vi "Alarm Settings.vi"(3 "Avg Temp Alarm On?":bool) -> (0 "Array of alarm limits":i32[](array[numeric]))   [LabVIEW 2014]
uses:
  <vilib>/Platform/TimedLoop/XDataNode/XDataNode.xnode
  <vilib>/Platform/TimedLoop/XDataNode/nitl_modes.ctl
  <vilib>/Platform/TimedLoop/XDataNode/XDNodeRunTimeDep.lvlib
  <vilib>/Platform/TimedLoop/XDataNode/wakeup.ctl
  <vilib>/Platform/TimedLoop/XDataNode/timing_clust.ctl
panel:
  in  "Max Spike":i32
  in  "Temperature Bounds High":i32
  in  "Temperature Bounds Low":i32
  # "Alarm Settings"
  # "Low"
  # "High"
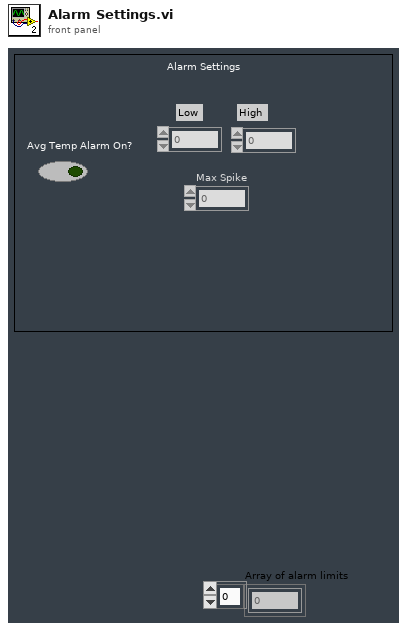
[diagram p1: front panel]
types:
  T1 = typedef "XDNodeRunTimeDep.lvlib/timing_clust.ctl" = cluster{"Expected End [f-1]":u64, "Actual End [f-1]":u64, "Finished Late? [f-1]":bool, "Expected End [i-1]":u64, "Actual End [i-1]":u64, "Finished Late? [i-1]":bool, "Expected Start [i]":u64, "Actual Start [i]":u64, "Expected Start [f]":u64, "Actual Start [f]":u64, "Source Name":string, "Structure Name":string, "Period":i64, "Deadline":i64, "Offset":i64, "Start":i64, "Priority":i32, "Timeout":i32, "Mode":T2, "Wakeup Reason":T3, "Error":errorcluster, "Source Type":string, "Secondary Source Type":string, "Global End Time":u64, "Global Start Time":u64, "Frame Duration":u64, "Iteration Duration":u64, "Assigned CPU":i32, "I/O Scan Engine Mode":u32}
  T2 = typedef "XDNodeRunTimeDep.lvlib/nitl_modes.ctl" = enum32{"No Change", "Process missed periods, maintain original phase", "Discard missed periods, maintain original phase", "Process missed periods, ignore original phase", "Discard missed periods, ignore original phase"}
  T3 = typedef "XDNodeRunTimeDep.lvlib/wakeup.ctl" = enum32{"Normal", "Aborted", "Asynchronous wakeup", "Timing source error", "Timed loop error", "Timeout"}
  T4 = enum8{"Enabled", "Disabled", "Disabled and Grayed Out"}
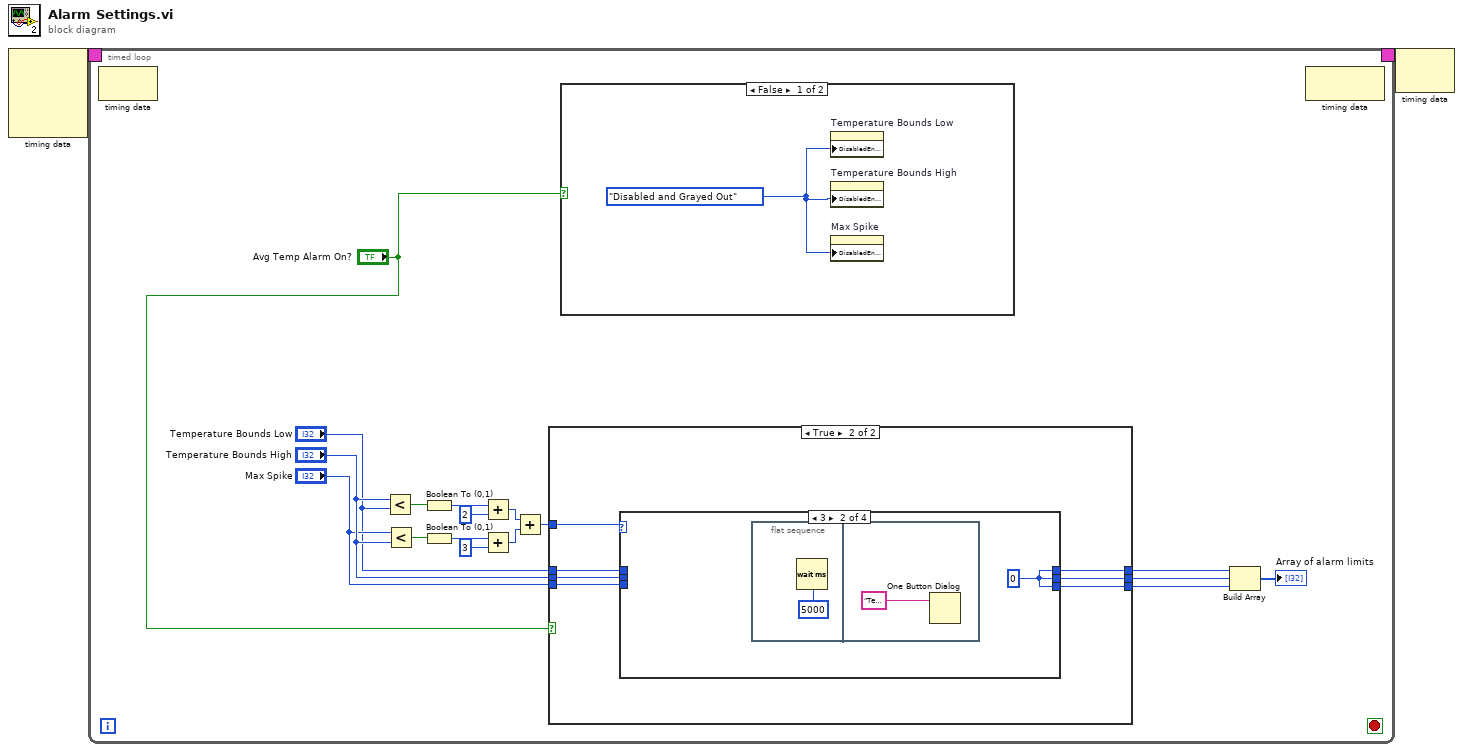
[diagram p0: block diagram]
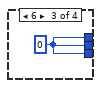
[diagram p4: hidden frame]
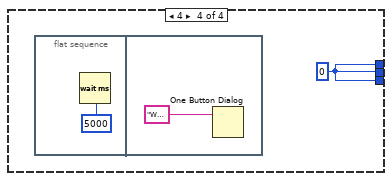
[diagram p5: hidden frame]
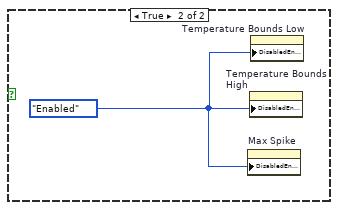
[diagram p6: hidden frame]
diagram:
  n1 = node-c288() -> (w2:T1)  [unwired: 4 in]
  n2 = timed-loop {
    timing: w2 -> [_]
    timing-out: [_] -> w1
    stop <- _ stop-if-true
    n3 = node-c288() -> ()  [unwired: 1 in, 1 out]
    n4 = Less?(x="Temperature Bounds High", y="Temperature Bounds Low") -> (x < y?=w16:bool)
    n5 = Less?(x="Max Spike", y="Temperature Bounds High") -> (x < y?=w11:bool)
    n6 = Boolean To (0,1)(Boolean=w16) -> (0, 1=w15:i16)
    n7 = Boolean To (0,1)(Boolean=w11) -> (0, 1=w13:i16)
    n8 = Add(x=w15, y=i16 2) -> (x+y=w9:i16)
    n9 = Add(x=w13, y=i16 3) -> (x+y=w10:i16)
    n10 = Add(x=w9, y=w10) -> (x+y=w8:i16)
    n11 = case shown="True" "Avg Temp Alarm On?" {
      tunnel: "Temperature Bounds High" -> [_ w22]
      tunnel: w8 -> [_ w26]
      tunnel: [_ w25] -> w7
      tunnel: [_ w24] -> w6
      tunnel: [_ w23] -> w5
      tunnel: "Max Spike" -> [_ w21]
      tunnel: "Temperature Bounds Low" -> [_ w20]
      frame False {
      }
      frame True {
        n12 = case shown="3" w26 {
          tunnel: [w27 w30 w33 w34] -> w25
          tunnel: [w29 w30 w33 w34] -> w24
          tunnel: [w28 w30 w33 w34] -> w23
          tunnel: w22 -> [w29 _ _ _]
          tunnel: w21 -> [w28 _ _ _]
          tunnel: w20 -> [w27 _ _ _]
          frame 5, Default {
          }
          frame 3 {
            w30 = 0 ("Temperature Bounds High")
            n13 = flat-sequence {
              frame #0 {
                n14 = Wait (ms)(milliseconds to wait=u32 5000) -> ()  [unwired: 1 out]
              }
              frame #1 {
                n15 = One Button Dialog(message="Temperature minimum higher than Temperature maximum!ARNING: Max Spike must be set higher than the Max Temperature Bounds!") -> ()  [unwired: 1 in, 1 out]
              }
            }
          }
          frame 6 {
            w33 = 0
          }
          frame 4 {
            w34 = 0 ("Temperature Bounds High")
            n16 = flat-sequence {
              frame #0 {
                n17 = Wait (ms)(milliseconds to wait=u32 5000) -> ()  [unwired: 1 out]
              }
              frame #1 {
                n18 = One Button Dialog(message="WARNING: Max Spike must be set higher than the Max Temperature Bounds!") -> ()  [unwired: 1 in, 1 out]
              }
            }
          }
        }
      }
    }
    n19 = case shown="False" "Avg Temp Alarm On?" {
      frame False {
        w39 = T4."Disabled and Grayed Out" ("Disabled")
        n20 = property on="Temperature Bounds Low" class="DigNum (strict)"("DisabledEnum"=w39) -> ()  [unwired: 2 in, 2 out]
        n21 = property on="Temperature Bounds High" class="DigNum (strict)"("DisabledEnum"=w39) -> ()  [unwired: 2 in, 2 out]
        n22 = property on="Max Spike" class="DigNum (strict)"("DisabledEnum"=w39) -> ()  [unwired: 2 in, 2 out]
      }
      frame True {
        w40 = T4."Enabled" ("Disabled")
        n23 = property on="Max Spike" class="DigNum (strict)"("DisabledEnum"=w40) -> ()  [unwired: 2 in, 2 out]
        n24 = property on="Temperature Bounds High" class="DigNum (strict)"("DisabledEnum"=w40) -> ()  [unwired: 2 in, 2 out]
        n25 = property on="Temperature Bounds Low" class="DigNum (strict)"("DisabledEnum"=w40) -> ()  [unwired: 2 in, 2 out]
      }
    }
    n26 = Build Array(w7, w6, w5) -> (→"Array of alarm limits":i32[])
    n27 = node-c288() -> ()  [unwired: 1 in, 1 out]
  }
  n28 = node-c288(w1) -> ()  [unwired: 1 out]
